vi "TestDynamixel.vi"() -> ()   [LabVIEW 2013]
uses:
  Data/TypeDefs/Sail Set Suggestions.ctl
  Data/TypeDefs/Rudder Set Suggestions.ctl
  Data/TypeDefs/MotorSetup.ctl
  Data/TypeDefs/DynamixelSetupInfo.ctl
  Data/TypeDefs/HardwareOnline.ctl
  Data/TypeDefs/DynamixelCycleTracker.ctl
  <instrlib>/Dynamixel Motor/Dynamixel Motor.lvlib
panel:
  out "Current Cycle State":T1
  in  "Motor Setup":T2
  out "Read Dynamixel positions":dbl[](array[numeric])
  out "Current Hardware Setup":T4
  out "Think Heartbeat":bool
  out "Sense Heartbeat":bool
  out "Act Heartbeat":bool
  out "Current Motor Setup":T2
  in  "Rudder Position Notifier":T5 min=-0.95 max=0.95 scale=1.0..-1.0
  in  "Sail Positions Notifier":T6 {"MainSailSuggestion" min=0.0 max=1.0; "JibSailSuggestion" min=0.0 max=1.0}
  out "Motors IDs Found":u8[](array[numeric])
  in  "stop":bool
  # "setting this to 360 if lower is 0 seems to trigger\ninfinite turning\nbut setting to 359 is OK"
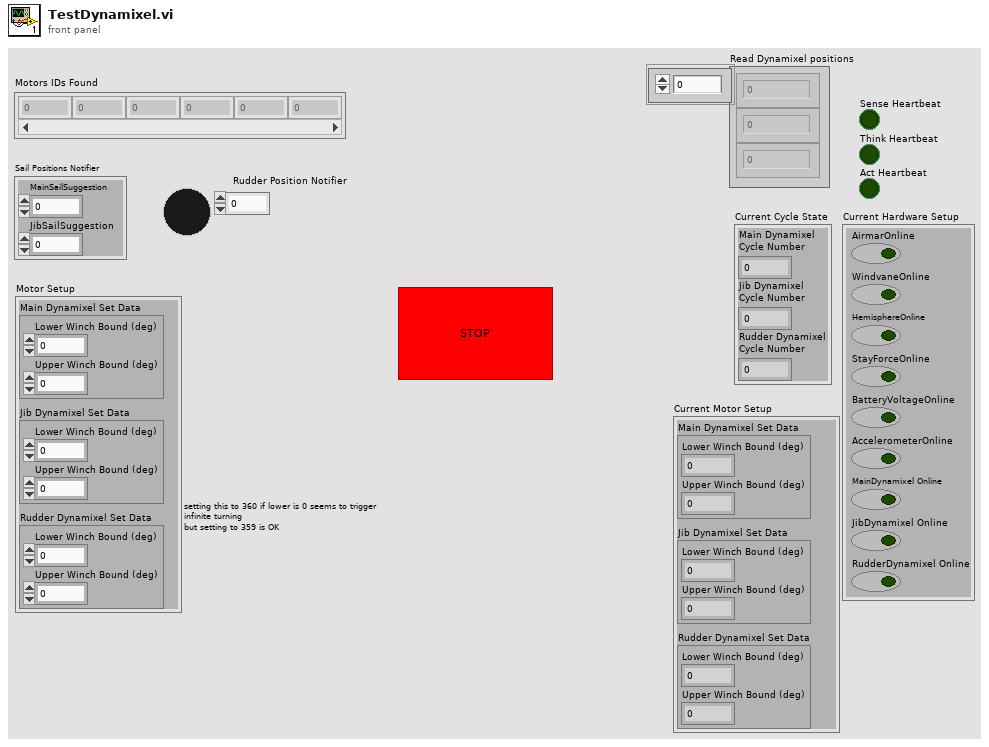
[diagram p1: front panel]
types:
  T1 = typedef "DynamixelCycleTracker.ctl" = cluster{"Main Dynamixel\nCycle Number":i32, "Jib Dynamixel\nCycle Number":i32, "Rudder Dynamixel\nCycle Number":i32}
  T2 = typedef "MotorSetup.ctl" = cluster{"Main Dynamixel Set Data":T3, "Rudder Dynamixel Set Data":T3, "Jib Dynamixel Set Data":T3}
  T3 = typedef "DynamixelSetupInfo.ctl" = cluster{"Lower Winch Bound (deg)":dbl, "Upper Winch Bound (deg)":dbl}
  T4 = typedef "HardwareOnline.ctl" = cluster{"AirmarOnline":bool, "WindvaneOnline":bool, "HemisphereOnline":bool, "StayForceOnline":bool, "BatteryVoltageOnline":bool, "AccelerometerOnline":bool, "MainDynamixel Online":bool, "JibDynamixel Online":bool, "RudderDynamixel Online":bool}
  T5 = typedef "Rudder Set Suggestions.ctl" = dbl
  T6 = typedef "Sail Set Suggestions.ctl" = cluster{"MainSailSuggestion":dbl, "JibSailSuggestion":dbl}
  T7 = enum16{"Blackbody Radiation", "Little boats", "Simulation", "Damn Yankee"}
  T8 = typedef "Notifiers.ctl" = cluster{"BoatSpeed":refnum<notifier>, "WindSpeed":refnum<notifier>, "EStop":refnum<notifier>, "BoatDirection":refnum<notifier>, "Luffing":refnum<notifier>, "RudderForce":refnum<notifier>, "BatteryVoltage":refnum<notifier>, "StayForces":refnum<notifier>, "BoatLocation":refnum<notifier>, "Pitch":refnum<notifier>, "Roll":refnum<notifier>, "RateOfTurn":refnum<notifier>, "RelWindDirection":refnum<notifier>, "SailPositions":refnum<notifier>, "RudderPosition":refnum<notifier>, "IronsRange":refnum<notifier>, "AbsWindDirection":refnum<notifier>, "OverrideInformation":refnum<notifier>, "DynamixelTorques":refnum<notifier>, "MotorSetup":refnum<notifier>, "AirmarStatus":refnum<notifier>, "HardwareOnline?":refnum<notifier>, "Sim_ActualSailPositions [0,1]":refnum<notifier>, "DynamixelCycleTracker":refnum<notifier>, "BoatVelocityDirection":refnum<notifier>, "SimWindHeading(rad)":refnum<notifier>, "SimWindSpeed(m/s)":refnum<notifier>, "RCInputValues":refnum<notifier>, "Finished Waypoints":refnum<notifier>, "DesiredHeading":refnum<notifier>, "Latest Mission ID":refnum<notifier>, "Latest Obstacle ID":refnum<notifier>, "DownwindDiscouragedRange":refnum<notifier>, "Tack Range":refnum<notifier>}
  T9 = typedef "GPS-Compass Queue Cluster.ctl" = cluster{"BoatLocation Queue":refnum<queue>, "BoatDirection Queue":refnum<queue>, "BoatSpeed Queue":refnum<queue>, "RateOfTurn Queue":refnum<queue>, "Pitch Queue":refnum<queue>, "Roll Queue":refnum<queue>, "BoatVelocityDirection Queue ":refnum<queue>}
  T10 = typedef "WindData Queue Cluster.ctl" = cluster{"RelWindDirection Queue":refnum<queue>, "WindSpeed Queue":refnum<queue>, "AbsWindDirection Queue":refnum<queue>}
  T11 = cluster{"Shroud Queue":refnum<queue>, "Battery Voltage Queue":refnum<queue>, "Accelerometer Queue":refnum<queue>, "AirmarGPS-Compass Queue Cluster":T9, "Hemisphere Queue Cluster":T9, "Airmar Wind Queue Cluster":T10, "Wind Vane Queue Cluster":T10, "Little Boat Queues":cluster{"Heading Queue":refnum<queue>, "Location Queue":refnum<queue>, "Wind Speed Queue":refnum<queue>, "Tilt Queue":refnum<queue>, "Wind Direction Queue":refnum<queue>}, "DynamixelTorque Queue":refnum<queue>, "DynamixelPosition Queue":refnum<queue>}
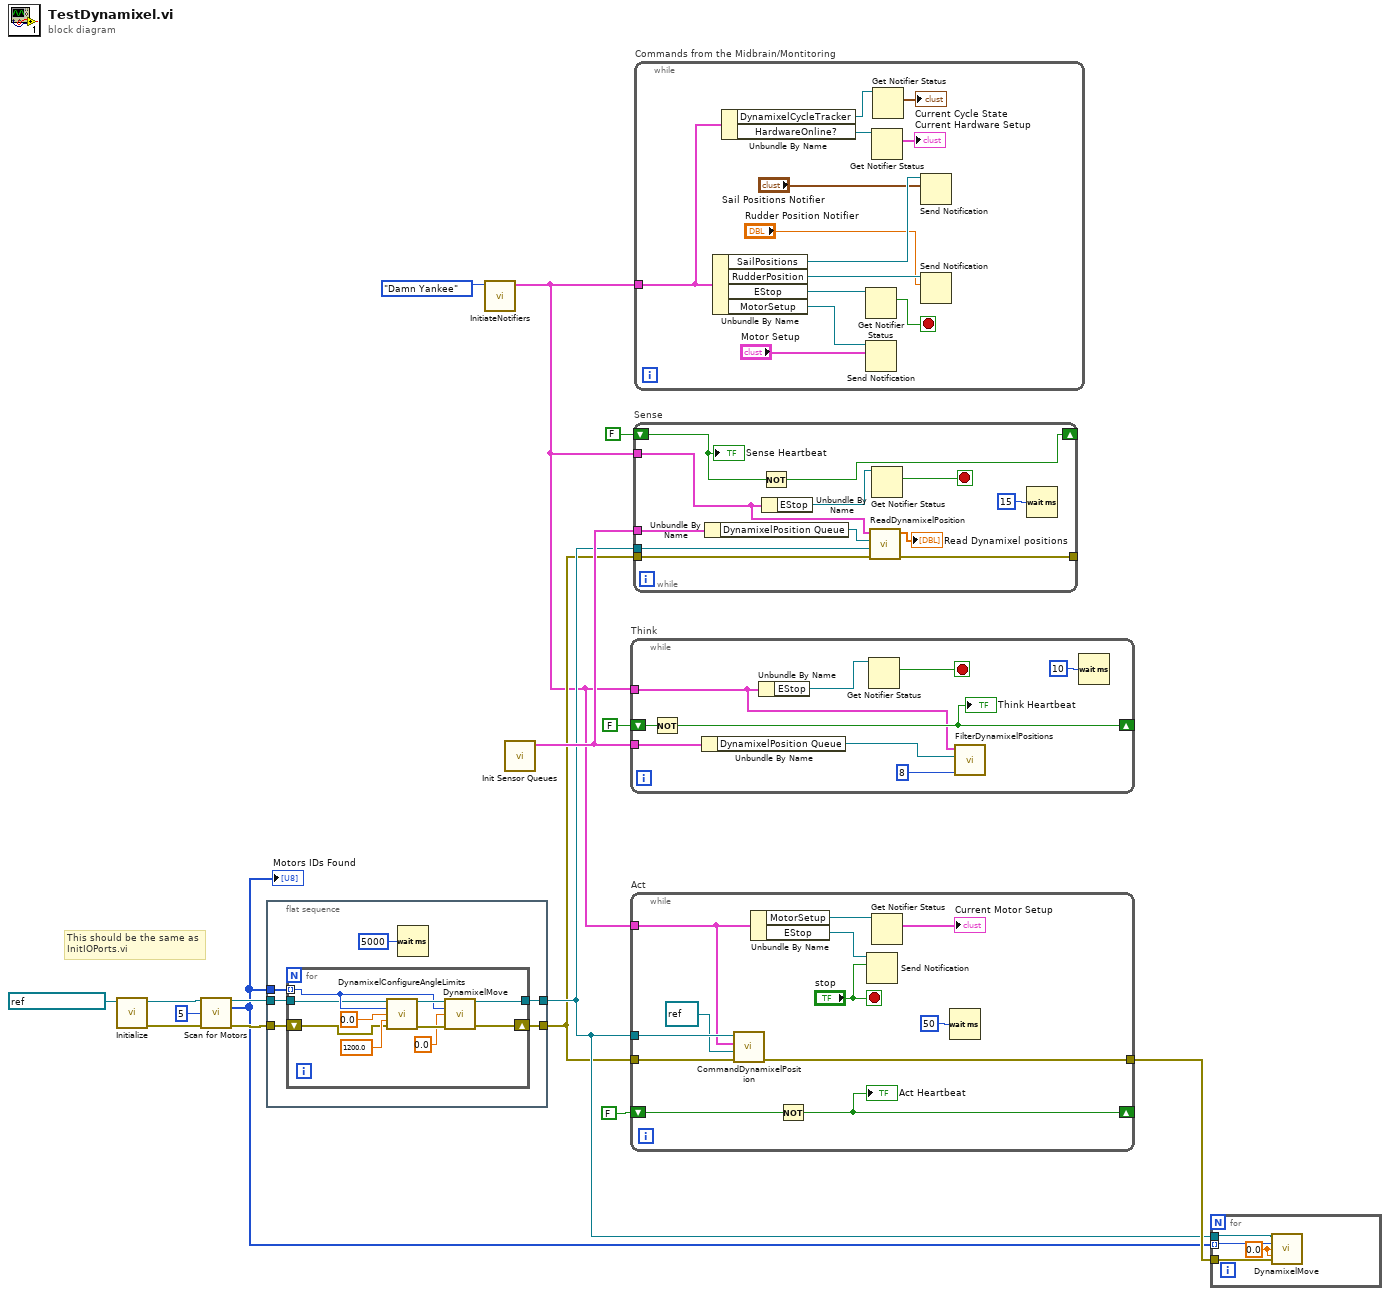
[diagram p0: block diagram]
diagram:
  # "This should be the same as InitIOPorts.vi"
  n1 = call <instrlib>:"Initialize.vi"("VISA resource name"=refnum<visa-resource-name> "ASRL3::INSTR") -> ("error out"=w13:errorcluster, "VISA resource name out"=w14:refnum<visa-resource-name>)  [unwired: 9 in]
  n2 = call <instrlib>:"Scan for Motors.vi"("VISA resource name"=w14, "Ending ID (253)"=u8 5, "error in (no error)"=w13) -> ("VISA resource name out"=w6:refnum<visa-resource-name>, "Motors IDs Found"=w2:u8[], "error out"=w4:errorcluster)  [unwired: 10 in]
  "Motors IDs Found" <- w2
  n3 = flat-sequence {
    tunnel: w6 -> [w20]
    tunnel: [w19] -> w5
    tunnel: w4 -> [w22]
    tunnel: [w21] -> w3
    tunnel: w2 -> [w18]
    frame #0 {
      n4 = for {
        shift-right: [w23] -> w21
        shift-left: w22 -> [w27]
        tunnel: w20 -> [w24]
        tunnel: [w25] -> w19
        tunnel: w18 -> [w28] mode=indexing
        n5 = call "DynamixelConfigureAngleLimits.vi"("VISA resource name"=w24, "Motor ID (0)"=w28, "Clockwise Angle Limit (0 deg)"=0.0, "Counter-Clockwise Angle Limit (300 deg)"=1200.0, "error in (no error)"=w27) -> ("VISA resource name out"=w31:refnum<visa-resource-name>, "error out"=w32:errorcluster)  [unwired: 9 in]
        n6 = call "DynamixelMove.vi"("VISA resource name"=w31, "Motor ID (0)"=w28, "Goal Position (150 deg)"=0.0, "error in (no error)"=w32) -> ("VISA resource name out"=w25:refnum<visa-resource-name>, "error out"=w23:errorcluster)  [unwired: 10 in]
      }
      n7 = Wait (ms)(milliseconds to wait=u32 5000) -> ()  [unwired: 1 out]
    }
  }
  n8 = call "InitiateNotifiers.vi"("Boat Type"=T7."Damn Yankee") -> ("NotifierReferences"=w1:T8)  [unwired: 8 in, 2 out]
  n9 = call "Init Sensor Queues.vi"() -> ("output cluster"=w11:T11)  [unwired: 11 in]
  n10 = while "Think" {
    tunnel: w1 -> [w33]
    tunnel: w11 -> [w41]
    shift-right: [w35] -> _
    shift-left: FALSE -> [w36]
    stop <- w37 stop-if-true
    n11 = Not(x=w36) -> (.not. x?=w35:bool)
    "Think Heartbeat" <- w35
    n12 = Unbundle By Name(w41) -> ("DynamixelPosition Queue"=w40:refnum<queue>)
    n13 = Unbundle By Name(w33) -> ("EStop"=w38:refnum<notifier>)
    n14 = Get Notifier Status(notifier=w38) -> (current notification=w37:bool)  [unwired: 1 in, 4 out]
    n15 = call "FilterDynamixelPositions.vi"("Queue timeout (ms)"=8, "DynamixelPosition Queue"=w40, "NotifierReff"=w33) -> ()  [unwired: 9 in]
    n16 = Wait (ms)(milliseconds to wait=u32 10) -> ()  [unwired: 1 out]
  }
  n17 = while "Act" {
    tunnel: w5 -> [w52]
    tunnel: w3 -> [w51]
    tunnel: w1 -> [w50]
    tunnel: [w45] -> w7
    shift-right: [w43] -> _
    shift-left: FALSE -> [w44]
    stop <- "stop" stop-if-true
    n18 = call "CommandDynamixelPosition.vi"("error in"=w51, "FPGA VI Reference In"=refnum<k20> refnum, "NotifierReff"=w50, "VISA resource name"=w52) -> ("Error out"=w45:errorcluster)  [unwired: 7 in]
    n19 = Unbundle By Name(w50) -> ("MotorSetup"=w47:refnum<notifier>, "EStop"=w49:refnum<notifier>)
    n20 = Not(x=w44) -> (.not. x?=w43:bool)
    "Act Heartbeat" <- w43
    n21 = Send Notification(notification="stop", notifier=w49) -> ()  [unwired: 1 in, 2 out]
    n22 = Get Notifier Status(notifier=w47) -> (current notification=→"Current Motor Setup":T2)  [unwired: 1 in, 4 out]
    n23 = Wait (ms)(milliseconds to wait=u32 50) -> ()  [unwired: 1 out]
  }
  n24 = while "Sense" {
    tunnel: w11 -> [w65]
    tunnel: w1 -> [w55]
    tunnel: w5 -> [w63]
    tunnel: w3 -> [w62]
    tunnel: [w61] -> _
    shift-right: [w58] -> _
    shift-left: FALSE -> [w57]
    stop <- w59 stop-if-true
    n25 = Unbundle By Name(w65) -> ("DynamixelPosition Queue"=w64:refnum<queue>)
    n26 = Not(x=w57) -> (.not. x?=w58:bool)
    n27 = Unbundle By Name(w55) -> ("EStop"=w60:refnum<notifier>)
    n28 = call "ReadDynamixelPosition.vi"("error in (no error)"=w62, "VISA resource name"=w63, "DynamixelPositions Queue"=w64, "Notifier References"=w55) -> ("error out"=w61:errorcluster, "Dynamixel positions"=→"Read Dynamixel positions":dbl[])  [unwired: 6 in]
    n29 = Get Notifier Status(notifier=w60) -> (current notification=w59:bool)  [unwired: 1 in, 4 out]
    n30 = Wait (ms)(milliseconds to wait=u32 15) -> ()  [unwired: 1 out]
    "Sense Heartbeat" <- w57
  }
  n31 = while "Commands from the Midbrain/Montitoring" {
    tunnel: w1 -> [w69]
    stop <- w77 stop-if-true
    n32 = Unbundle By Name(w69) -> ("SailPositions"=w76:refnum<notifier>, "RudderPosition"=w75:refnum<notifier>, "EStop"=w78:refnum<notifier>, "MotorSetup"=w72:refnum<notifier>)
    n33 = Unbundle By Name(w69) -> ("DynamixelCycleTracker"=w67:refnum<notifier>, "HardwareOnline?"=w68:refnum<notifier>)
    n34 = Get Notifier Status(notifier=w78) -> (current notification=w77:bool)  [unwired: 1 in, 4 out]
    n35 = Send Notification(notification="Motor Setup", notifier=w72) -> ()  [unwired: 1 in, 2 out]
    n36 = Get Notifier Status(notifier=w68) -> (current notification=→"Current Hardware Setup":T4)  [unwired: 1 in, 4 out]
    n37 = Get Notifier Status(notifier=w67) -> (current notification=→"Current Cycle State":T1)  [unwired: 1 in, 4 out]
    n38 = Send Notification(notification="Sail Positions Notifier", notifier=w76) -> ()  [unwired: 1 in, 2 out]
    n39 = Send Notification(notification="Rudder Position Notifier", notifier=w75) -> ()  [unwired: 1 in, 2 out]
  }
  n40 = for {
    tunnel: w5 -> [w82]
    tunnel: w7 -> [w81]
    tunnel: w2 -> [w80] mode=indexing
    w79 = 0.0 ("Goal Position (150 deg)")
    n41 = call "DynamixelMove.vi"("VISA resource name"=w82, "Motor ID (0)"=w80, "Goal Position (150 deg)"=w79, "Goal Speed (RPM)"=w79, "error in (no error)"=w81) -> ()  [unwired: 9 in, 2 out]
  }
